vi "Set Spectrum Setup API.vi"(8 "Error In":errorcluster) -> (0 "Error Out":errorcluster)   [LabVIEW 2017, in "Main controller.lvlib"]
uses:
  Main controller.lvlib
  CTLs/Command Data [cluster].ctl
  CTLs/Commands [enum].ctl
  Events/Events.lvlib
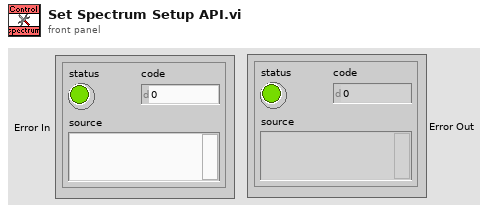
[diagram p1: front panel]
types:
  T1 = typedef "Main controller.lvlib/Command Data [cluster].ctl" = cluster{"Command":T2, "Data":variant}
  T2 = typedef "Main controller.lvlib/Commands [enum].ctl" = enum16{"Start", "Initialise Devices", "Stop", "Set DAQ data", "Set Scope data", "Set Spectrum Setup", "Spectrum Setup Complete", "Set Monochromator Setup", "Monochromator Setup Complete", "Set Monochromator data", "Set Colour Wheel Setup", "Colour Wheel Setup Complete", "Move Shutter", "Move Shutter Complete", "Collect Data", "DAQ Acquisition Complete", "Scope Acquisition Complete", "Collect Data Complete", "A-B Processing", "A-B Processing Complete", "DAQ-Scope Stitching", "DAQ-Scope Stitching Complete", "Return Shutter", "Return Shutter Complete", "Set colour wheel data", "Set all config data", "Acquire test data", "Accumulate test data", "Average test data", "All Averaging Complete", "DAQ Averaging Complete", "Scope Averaging Complete", "Finalise test data", "All Finalising Complete", "DAQ Finalising Complete", "Scope Finalising Complete", "Process test data", "End Test"}
  T3 = typedef "Events.lvlib/Refs [cluster].ctl" = cluster{"Exit":refnum<user-event>, "Controller":refnum<user-event>, "System Error":refnum<user-event>, "UI":refnum<user-event>, "Example Module":refnum<user-event>, "Shutter":refnum<user-event>, "Monochromator":refnum<user-event>, "DAQ":refnum<user-event>, "Scope":refnum<user-event>, "Processing":refnum<user-event>, "File IO":refnum<user-event>, "Colour wheel":refnum<user-event>}
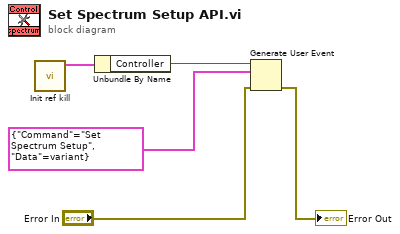
[diagram p0: block diagram]
diagram:
  n1 = call "Init ref kill.vi"() -> ("Messages"=w5:T3)  [unwired: 10 in, 1 out]
  n2 = Unbundle By Name(w5) -> ("Controller"=w4:refnum<user-event>)
  n3 = Generate User Event(user event=w4, event data cluster=T1 {"Command"=enum."Set Spectrum Setup", "Data"=variant} ("event data"), error in="Error In") -> (error out=→"Error Out":errorcluster)  [unwired: 1 in, 1 out]
